vi "GrabImages.vi"() -> (0 "Training Instructions":picture, 1 "Intro":picture, 2 "Table":picture, 3 "View Instructions":picture)   [LabVIEW 2021]
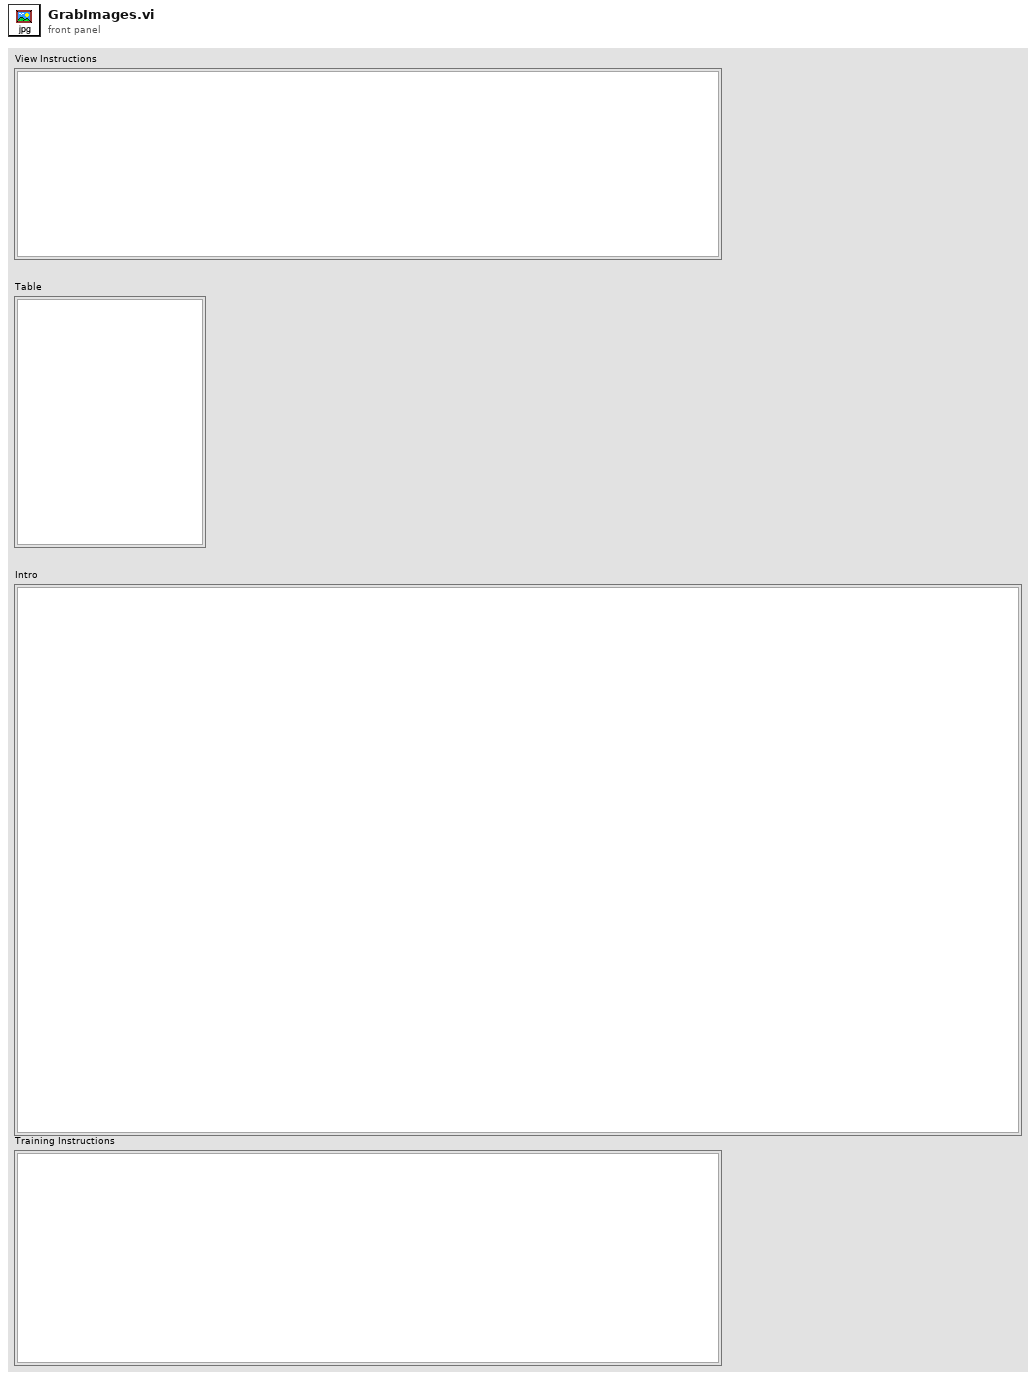
[diagram p1: front panel]
types:
  T1 = typedef "imagedata.ctl" = cluster{"image type":i32, "image depth":i32, "image":u8[], "mask":u8[], "colors":u32[], "Rectangle":cluster{"left":i16, "top":i16, "right":i16, "bottom":i16}}
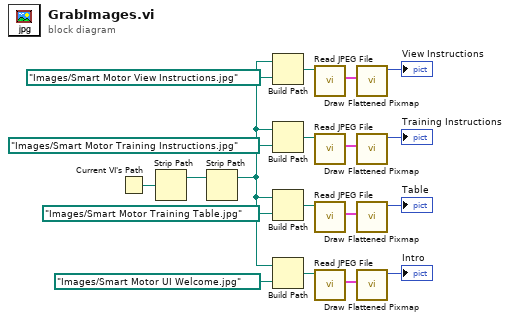
[diagram p0: block diagram]
diagram:
  n1 = Current VI's Path() -> (path=w3:path)
  n2 = Strip Path(path=w3) -> (stripped path=w2:path)  [unwired: 1 out]
  n3 = Strip Path(path=w2) -> (stripped path=w1:path)  [unwired: 1 out]
  n4 = Build Path(base path=w1, name or relative path=path "Images/Smart Motor View Instructions.jpg" ("path to JPEG file")) -> (appended path=w11:path)
  n5 = Build Path(base path=w1, name or relative path=path "Images/Smart Motor Training Instructions.jpg" ("path to JPEG file")) -> (appended path=w9:path)
  n6 = Build Path(base path=w1, name or relative path=path "Images/Smart Motor Training Table.jpg" ("path to JPEG file")) -> (appended path=w7:path)
  n7 = Build Path(base path=w1, name or relative path=path "Images/Smart Motor UI Welcome.jpg" ("path to JPEG file")) -> (appended path=w5:path)
  n8 = call <vilib>:"Read JPEG File.vi"("path to JPEG file"=w11) -> ("image data"=w13:T1)  [unwired: 8 in, 2 out]
  n9 = call <vilib>:"Read JPEG File.vi"("path to JPEG file"=w9) -> ("image data"=w19:T1)  [unwired: 8 in, 2 out]
  n10 = call <vilib>:"Read JPEG File.vi"("path to JPEG file"=w7) -> ("image data"=w17:T1)  [unwired: 8 in, 2 out]
  n11 = call <vilib>:"Read JPEG File.vi"("path to JPEG file"=w5) -> ("image data"=w15:T1)  [unwired: 8 in, 2 out]
  n12 = call <vilib>:"Draw Flattened Pixmap.vi"("image data"=w13) -> ("new picture"=→"View Instructions":picture)  [unwired: 8 in]
  n13 = call <vilib>:"Draw Flattened Pixmap.vi"("image data"=w19) -> ("new picture"=→"Training Instructions":picture)  [unwired: 8 in]
  n14 = call <vilib>:"Draw Flattened Pixmap.vi"("image data"=w17) -> ("new picture"=→"Table":picture)  [unwired: 8 in]
  n15 = call <vilib>:"Draw Flattened Pixmap.vi"("image data"=w15) -> ("new picture"=→"Intro":picture)  [unwired: 8 in]
